vi "Brute Force Dark Current Primary Logic Body.vi"(0 "Barcodes in":string[](array[string]), 1 "stop":bool, 2 "Pins In":refnum<k21>[](array[refnum]), 5 "VISA Refnum in":refnum<visa-resource-name>, 6 "Number of Tubes":i32, 7 "Channel #":i32) -> (10 "Actual Voltage Level (V)":dbl format="%#_13g", 11 "Individual Tube Current (Nano Amps)":dbl[](array[numeric]), 12 "Actual Current Limit (nA)":dbl format="%#_13g", 13 "Mesurnment Iteration":i32, 14 "Power Supply Trip":bool, 16 "Pins Out":refnum<k21>[](array[refnum]), 19 "Failed Tubes":string[](array[string]))   [LabVIEW 2020]
uses:
  <instrlib>/CAEN PSM/CAEN PSM.lvlib
panel:
  out "error out":errorcluster
  in  "First Tube #":i32
  out "BoardHandle out":T1
  # "Pin in"
  # "Pin out"
  # "No pin"
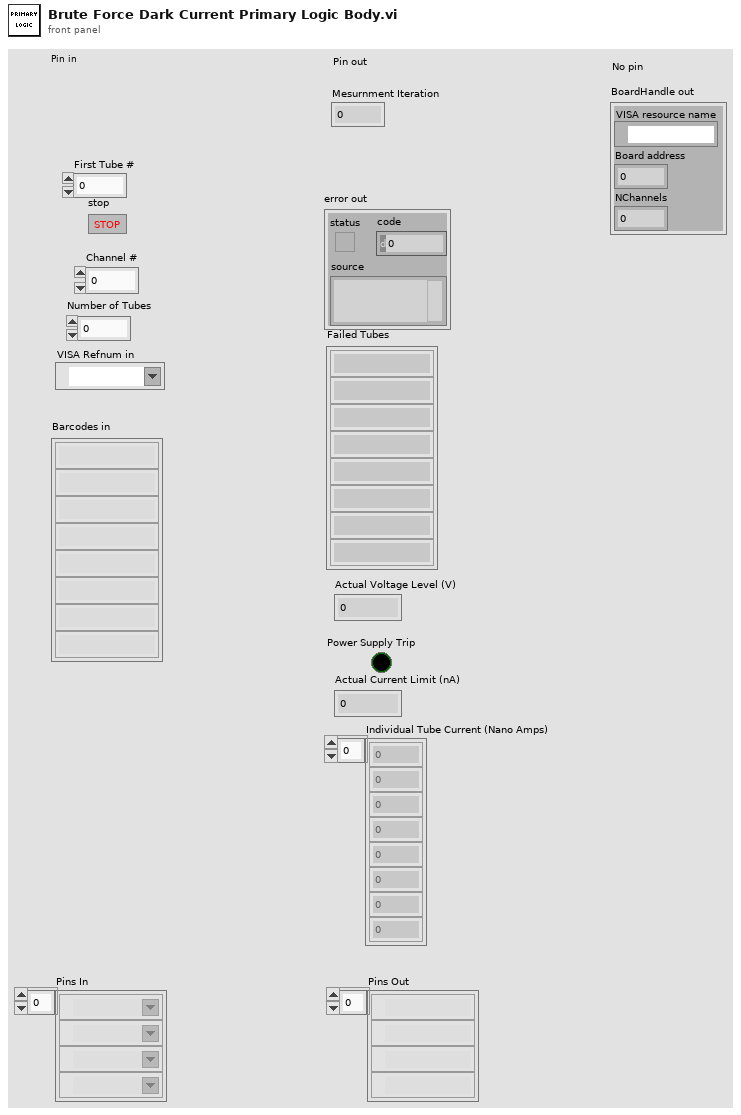
[diagram p1: front panel]
types:
  T1 = cluster{"VISA resource name":refnum<visa-resource-name>, "Board address":u8, "NChannels":u8}
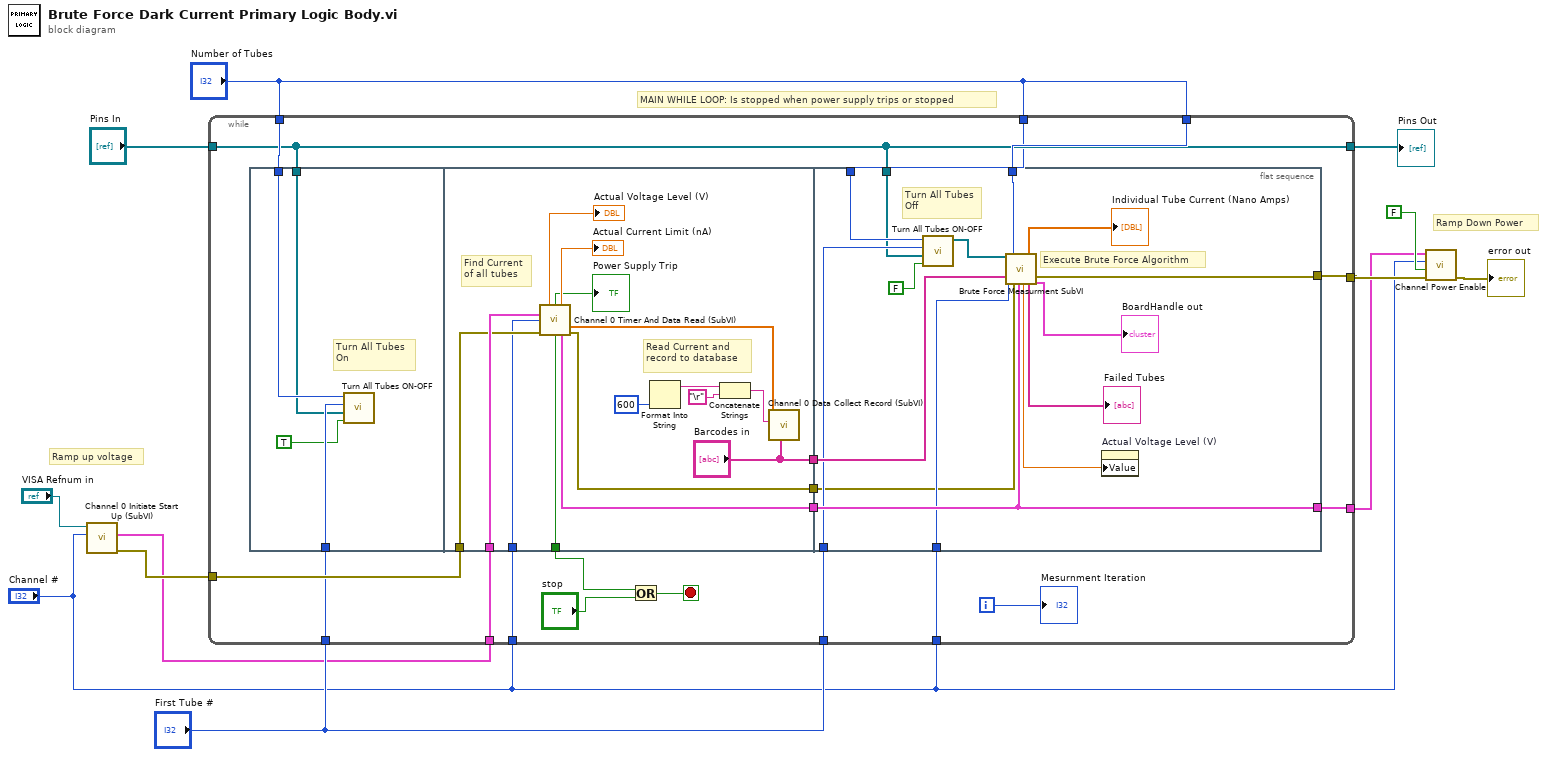
[diagram p0: block diagram]
diagram:
  # "Ramp Down Power"
  # "MAIN WHILE LOOP: Is stopped when power supply trips or stopped"
  # "Ramp up voltage"
  n1 = call "Channel 0 Initiate Start Up (SubVI).vi"("Channel # in"="Channel #", "VISA Refnum in"="VISA Refnum in") -> ("error out"=w7:errorcluster, "BoardHandle out"=w6:T1)  [unwired: 8 in]
  n2 = while {
    tunnel: "Number of Tubes" -> [w31]
    tunnel: "First Tube #" -> [w30]
    tunnel: "Number of Tubes" -> [w13]
    tunnel: "Channel #" -> [w29]
    tunnel: w6 -> [w28]
    tunnel: "Number of Tubes" -> [w27]
    tunnel: w7 -> [w23]
    tunnel: "First Tube #" -> [w19]
    tunnel: [w17] -> w9
    tunnel: [w16] -> w11
    tunnel: "Pins In" -> [w14]
    tunnel: "Channel #" -> [w15]
    tunnel: [w14] -> w2
    i -> [w20]
    stop <- w21 stop-if-true
    n3 = flat-sequence {
      tunnel: w27 -> [w35]
      tunnel: w19 -> [w34]
      tunnel: w14 -> [w32]
      tunnel: w29 -> [w38]
      tunnel: w28 -> [w41]
      tunnel: [w45] -> w26
      tunnel: [w43] -> w25
      tunnel: ["Barcodes in"] -> w24
      tunnel: w23 -> [w40]
      tunnel: [w37] -> w22
      tunnel: w31 -> [w63]
      tunnel: w24 -> [w64]
      tunnel: w25 -> [w62]
      tunnel: w26 -> [w52]
      tunnel: w13 -> [w57]
      tunnel: w30 -> [w56]
      tunnel: [w62] -> w17
      tunnel: [w51] -> w16
      tunnel: w15 -> [w54]
      tunnel: w14 -> [w53]
      frame #0 {
        # "Turn All Tubes \nOn"
        n4 = call "Turn All Tubes ON-OFF.vi"("Activate: 1\nDeactivate: 0"=TRUE, "Pins In"=w32, "First Tube #"=w34, "Last Tube #"=w35) -> ()  [unwired: 7 in, 1 out]
      }
      frame #1 {
        # "Find Current\nof all tubes"
        # "Read Current and  record to database"
        n5 = call "Channel 0 Timer And Data Read (SubVI).vi"("BoardHandle in"=w41, "Channel # in"=w38, "error in (no error)"=w40) -> ("Actual Voltage Level (V)"=→"Actual Voltage Level (V)":dbl, "Power Supply Trip"=w37:bool, "Actual Current Limit (nA)"=→"Actual Current Limit (nA)":dbl, "Array"=w44:dbl[], "BoardHandle out 2"=w43:T1, "error out"=w45:errorcluster)  [unwired: 7 in]
        "Power Supply Trip" <- w37
        n6 = Format Into String(600 ("input 1")) -> (resulting string=w48:string)  [unwired: 3 in, 1 out]
        n7 = Concatenate Strings(w48, "\r") -> (w49:string)
        n8 = call "Channel 0 Data Collect Record (SubVI).vi"("Barcodes"="Barcodes in", "Array"=w44, "String"=w49) -> ()  [unwired: 9 in]
      }
      frame #2 {
        # "Execute Brute Force Algorithm"
        # "Turn All Tubes\nOff"
        n9 = call "Turn All Tubes ON-OFF.vi"("Activate: 1\nDeactivate: 0"=FALSE ("Activate: 1\nDeactivate: 0"), "Pins In"=w53, "First Tube #"=w56, "Last Tube #"=w57) -> ("Pins Out"=w50:refnum<k21>[])  [unwired: 7 in]
        n10 = call "Brute Force Measurment SubVI.vi"("Pins In"=w50, "Barcodes in"=w64, "Channel # in"=w54, "Last Tube #"=w63, "error in (no error)"=w52, "BoardHandle in"=w62) -> ("Actual Voltage Level (V) 2"=w61:dbl, "Individual Tube Current (Nano Amps)"=→"Individual Tube Current (Nano Amps)":dbl[], "Failed Tubes"=→"Failed Tubes":string[], "error out"=w51:errorcluster, "BoardHandle out"=→"BoardHandle out":T1)  [unwired: 8 in, 1 out]
        n11 = property on="Actual Voltage Level (V)" class="DigNum (strict)"("Value"=w61) -> ()  [unwired: 2 in, 2 out]
      }
    }
    n12 = Or(x=w22, y="stop") -> (x .or. y?=w21:bool)
    "Mesurnment Iteration" <- w20
  }
  "Pins Out" <- w2
  n13 = call <instrlib>:"Channel Power Enable.vi"("error in (no error)"=w11, "Enable (OFF)"=FALSE, "Channel (0)"="Channel #", "BoardHandle"=w9) -> ("error out"=→"error out":errorcluster)  [unwired: 6 in, 1 out]
